vi "closeEventReferences.vi"(8 "error in (no error)":errorcluster, 11 "ViewThisComponent in":refnum<class "ViewThisComponent.lvclass">) -> (0 "error out":errorcluster, 3 "ViewThisComponent out":refnum<class "ViewThisComponent.lvclass">)   [LabVIEW 2015, in "ViewThisComponent.lvclass"]
uses:
  ViewThisComponent.lvclass
  ViewThisComponent.lvclass/ViewThisComponent.ctl
  ComponentTemplateCore/ComponentModel/ComponentModel/View/View.lvclass
  PubSubDataEvent/PubSubDataEvent.lvclass
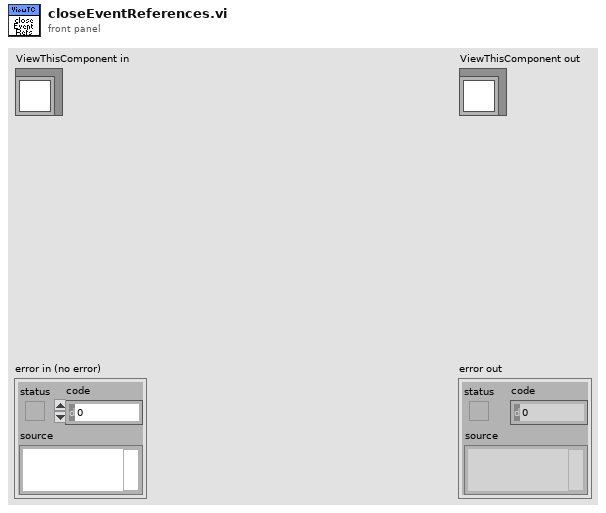
[diagram p1: front panel]
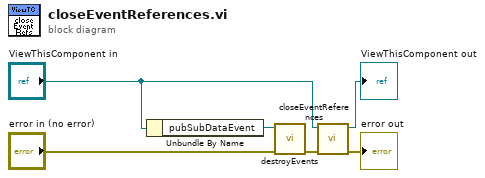
[diagram p0: block diagram]
diagram:
  n1 = Unbundle By Name("ViewThisComponent in") -> ("pubSubDataEvent"=w4:refnum<class "PubSubDataEvent.lvclass">)
  n2 = call "destroyEvents.vi"("error in (no error)"="error in (no error)", "PubSubDataEvent in"=w4) -> ("error out"=w2:errorcluster)  [unwired: 8 in, 1 out]
  n3 = call-parent "closeEventReferences.vi"("error in (no error)"=w2, "View in"="ViewThisComponent in") -> ("error out"=→"error out":errorcluster, "View out"=→"ViewThisComponent out":refnum<class "ViewThisComponent.lvclass">)  [unwired: 8 in]
